vi "StartExecutionCallback1.vi"(4 "Tab Control":refnum<vi>, 5 "Event Data":T1, 6 "Control Ref":refnum<k7>, 7 "Event Common Data":T2) -> ()   [LabVIEW 2009]
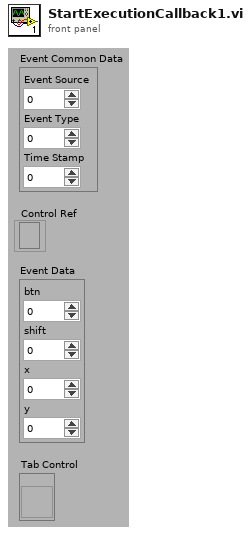
[diagram p1: front panel]
types:
  T1 = cluster{"btn":i16, "shift":i16, "x":i32, "y":i32}
  T2 = cluster{"Event Source":i32, "Event Type":u32, "Time Stamp":u32}
  T3 = enum32{"Test Sequence Builder", "Sequence Viewer", "Sequence Execution"}
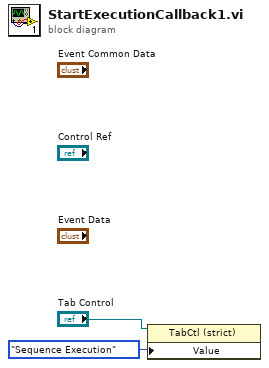
[diagram p0: block diagram]
diagram:
  n1 = property class="TabCtl (strict)"(reference="Tab Control", "Value"=T3."Sequence Execution") -> ()  [unwired: 1 in, 2 out]
